vi "fgv_DWA_process-val.vi"(7 "cmd":T2, 11 "prcess val":T1) -> (3 "prcess val out":T1)   [LabVIEW 2019]
uses:
  Ctrl/cmd_common.ctl
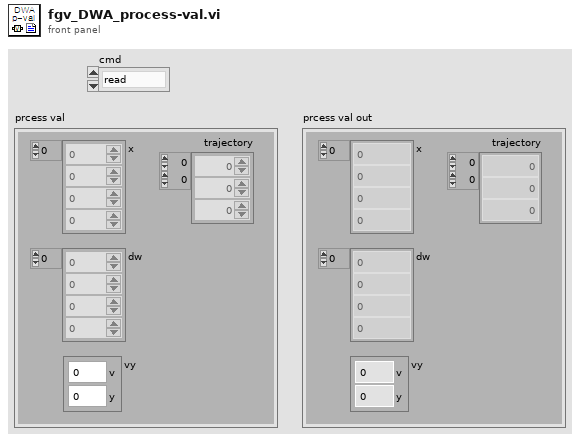
[diagram p1: front panel]
types:
  T1 = cluster{"x":dbl[], "dw":dbl[], "vy":cluster{"v":dbl, "y":dbl}, "trajectory":dbl[][]}
  T2 = typedef "cmd_common.ctl" = enum16{"read", "write"}
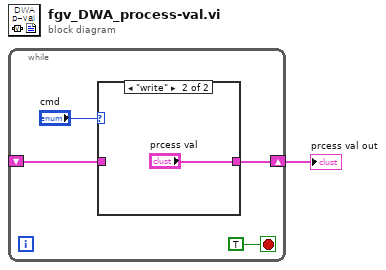
[diagram p0: block diagram]
diagram:
  n1 = while {
    shift-right: [w3] -> w1
    shift-left: _ -> [w2]
    stop <- TRUE stop-if-true
    n2 = case shown="\"write\"" "cmd" {
      tunnel: [w6 "prcess val"] -> w3
      tunnel: w2 -> [w6 _]
      frame "read", Default {
      }
      frame "write" {
      }
    }
  }
  "prcess val out" <- w1
